vi "Set Defaults from Strings.vi"(8 "error in (no error)":errorcluster, 10 "Default Strings":string[](array[string]), 11 "Group BOOL in":refnum<class "Group BOOL.lvclass">) -> (0 "error out":errorcluster, 3 "Group BOOL out":refnum<class "Group BOOL.lvclass">)   [LabVIEW 2020, in "Vecto.lvlib" / "Group BOOL.lvclass"]
uses:
  Group BOOL.lvclass
  Group BOOL.lvclass/Group BOOL.ctl
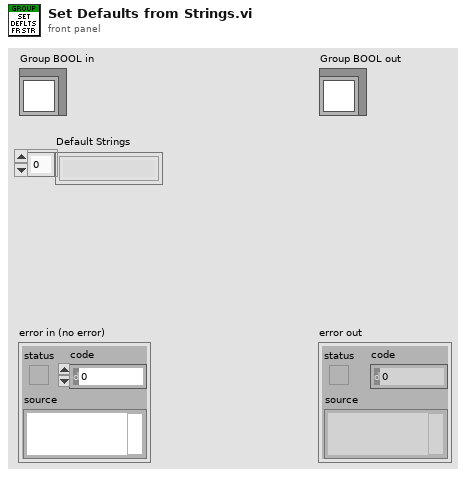
[diagram p1: front panel]
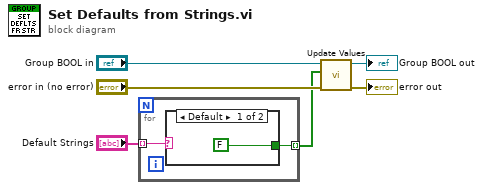
[diagram p0: block diagram]
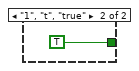
[diagram p2: hidden frame]
diagram:
  n1 = for {
    tunnel: "Default Strings" -> [w8] mode=indexing
    tunnel: [w7] -> w1 mode=indexing
    n2 = case shown="Default" w8 {
      tunnel: [FALSE TRUE] -> w7
      frame Default {
      }
      frame "1", "t", "true" {
      }
    }
  }
  n3 = call "Update Values.vi"("error in (no error)"="error in (no error)", "Values"=w1, "Group BOOL in"="Group BOOL in") -> ("error out"=→"error out":errorcluster, "Group BOOL out"=→"Group BOOL out":refnum<class "Group BOOL.lvclass">)  [unwired: 7 in]
